vi "Do Get Object Help.vi"(8 "error in (no error)":errorcluster, 10 "get_object_help Argument":T2, 11 "Data Cluster in":T1) -> (0 "error out":errorcluster, 2 "help_string":string, 3 "Data Cluster out":T1)   [LabVIEW 2025, in "Scripting Server.lvlib"]
uses:
  Scripting Server.lvlib
  get_object_help (Reply Payload)--cluster.ctl
  get_object_help Argument--cluster.ctl
  Module Data--cluster.ctl
panel:
  out "help tag":string
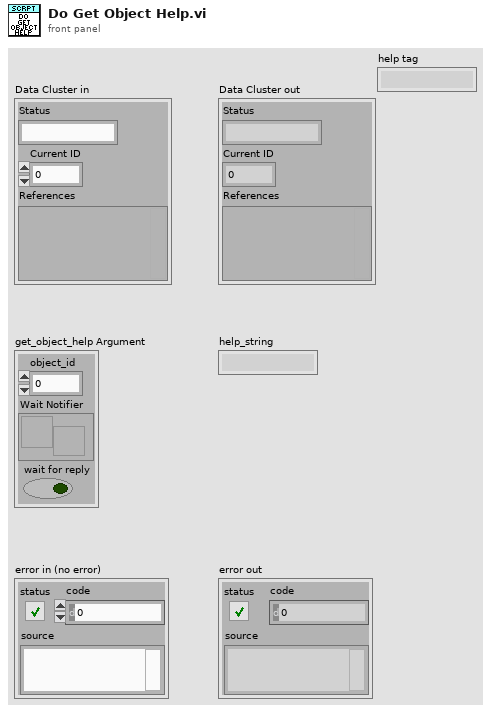
[diagram p1: front panel]
types:
  T1 = typedef "Scripting Server.lvlib/Module Data--cluster.ctl" = cluster{"Status":string, "Current ID":i32, "References":variant}
  T2 = typedef "Scripting Server.lvlib/get_object_help Argument--cluster.ctl" = cluster{"object_id":i32, "Wait Notifier":refnum<notifier>, "wait for reply":bool}
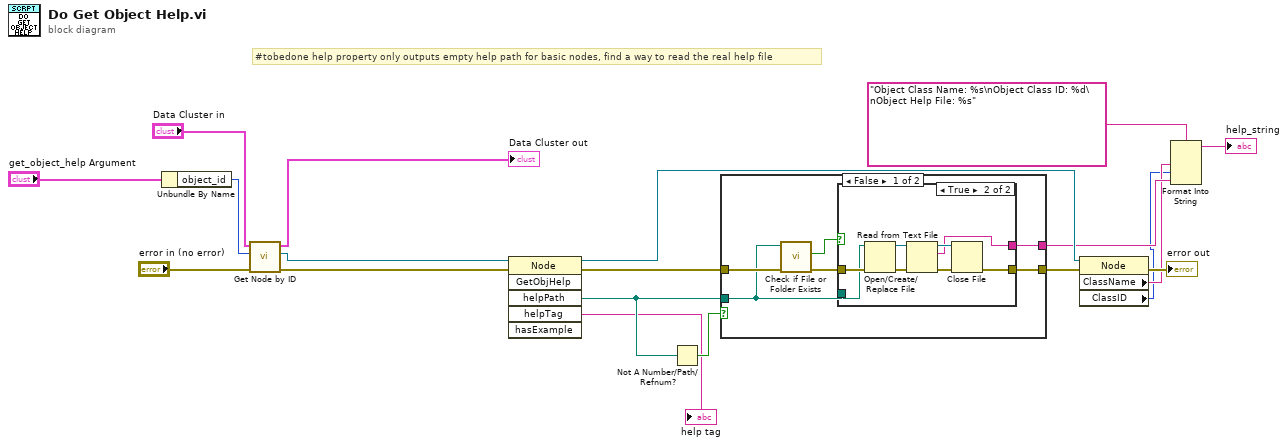
[diagram p0: block diagram]
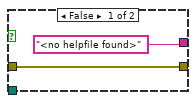
[diagram p2: hidden frame]
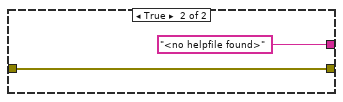
[diagram p3: hidden frame]
diagram:
  # "#tobedone help property only outputs empty help path for basic nodes, find a way to read the real help file"
  n1 = Unbundle By Name("get_object_help Argument") -> ("object_id"=w14:i32)
  n2 = call "Get Node by ID.vi"("error in (no error)"="error in (no error)", "ID"=w14, "Data Cluster in"="Data Cluster in") -> ("error out"=w17:errorcluster, "specific class reference"=w1:refnum<vi>, "Data Cluster out"=→"Data Cluster out":T1)  [unwired: 6 in]
  n3 = invoke class="Node" method="GetObjHelp"(reference=w1, error in=w17) -> (reference out=w11:refnum<vi>, error out=w12:errorcluster, "helpPath"=w8:path, "helpTag"=→"help tag":string)  [unwired: 4 in, 2 out]
  n4 = Not A Number/Path/Refnum?(number/path/refnum=w8) -> (NaN/Path/Refnum?=w9:bool)
  n5 = case shown="False" w9 {
    tunnel: w12 -> [w25 w37]
    tunnel: [w24 w37] -> w10
    tunnel: w8 -> [w21 _]
    tunnel: [w23 "<no helpfile found>"] -> w5
    frame False {
      n6 = call <vilib>:"Check if File or Folder Exists.vi"("error in (no error)"=w25, "path"=w21) -> ("error out"=w22:errorcluster, "file or folder exists?"=w20:bool)  [unwired: 7 in, 1 out]
      n7 = case shown="True" w20 {
        tunnel: [w27 w33] -> w24
        tunnel: ["<no helpfile found>" w30] -> w23
        tunnel: w22 -> [w27 w29]
        tunnel: w21 -> [_ w28]
        frame False {
        }
        frame True {
          n8 = Open/Create/Replace File(file path (use dialog)=w28, error in=w29) -> (refnum out=w32:refnum<file>, error out=w35:errorcluster)  [unwired: 4 in, 1 out]
          n9 = Read from Text File(file (use dialog)=w32, error in=w35) -> (refnum out=w31:refnum<file>, text=w30:string, error out=w34:errorcluster)  [unwired: 2 in, 1 out]
          n10 = Close File(refnum=w31, error in=w34) -> (error out=w33:errorcluster)  [unwired: 1 out]
        }
      }
    }
    frame True {
    }
  }
  n11 = property class="Node"(reference=w11, error in=w10) -> (error out=→"error out":errorcluster, "ClassName"=w4:string, "ClassID"=w3:u32)  [unwired: 1 out]
  n12 = Format Into String(format string="Object Class Name: %s\nObject Class ID: %d\nObject Help File: %s", w4, w3, w5) -> (resulting string=→"help_string":string)  [unwired: 2 in, 1 out]
